vi "Check folder &Create.vi"(7 "Boolean":bool=TRUE, 8 "error in (no error)":errorcluster, 9 "pattern":string, 10 "file name":string, 11 "folder name":string) -> (0 "error out":errorcluster, 3 "build path":path)   [LabVIEW 2010]
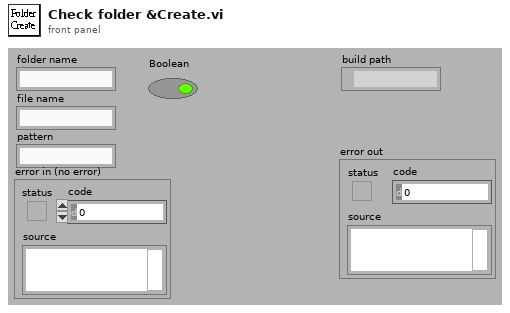
[diagram p1: front panel]
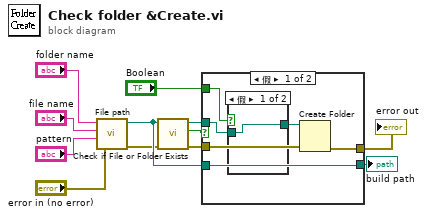
[diagram p0: block diagram]
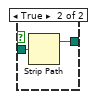
[diagram p2: hidden frame]
diagram:
  n1 = call "File path.vi"("folder name"="folder name", "file name"="file name", "pattern"="pattern", "error in (no error)"="error in (no error)") -> ("build path"=w11:path, "error out"=w8:errorcluster)  [unwired: 3 out]
  n2 = call <vilib>:"Check if File or Folder Exists.vi"("error in (no error)"=w8, "path"=w11) -> ("error out"=w12:errorcluster, "file or folder exists?"=w9:bool, "dup path"=w10:path)  [unwired: 7 in]
  n3 = case shown="假" w9 {
    tunnel: w10 -> [w18 _]
    tunnel: w11 -> [w17 w23]
    tunnel: [w17 w23] -> w3
    tunnel: w12 -> [w16 w22]
    tunnel: [w15 w22] -> w2
    tunnel: "Boolean" -> [w13 _]
    frame False {
      n4 = case shown="假" w13 {
        tunnel: w18 -> [w19 w21]
        tunnel: [w19 w20] -> w14
        frame False {
        }
        frame True {
          n5 = Strip Path(path=w21) -> (stripped path=w20:path)  [unwired: 1 out]
        }
      }
      n6 = Create Folder(path (use dialog)=w14, error in=w16) -> (error out=w15:errorcluster)  [unwired: 1 in, 2 out]
    }
    frame True {
    }
  }
  "build path" <- w3
  "error out" <- w2
